vi "HighPressureVerification.vi"(8 "error in":errorcluster, 11 "S1 in":refnum<class "S1.lvclass">) -> (0 "error out":errorcluster, 3 "S1 out":refnum<class "S1.lvclass">)   [LabVIEW 2018, in "S1.lvclass"]
uses:
  S1.lvclass
  S1.lvclass/S1.ctl
  Public Controls/Outputs.ctl
  Public Controls/ReportHeader.ctl
  d2b88b60-9070-42d4-a245-a35bcc0db904.vi
  8c384891-5d03-4ede-b955-697cfc4dec26.vi
  IO/IO.lvclass
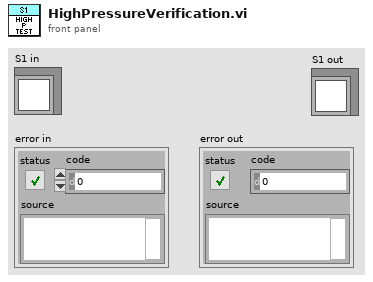
[diagram p1: front panel]
types:
  T1 = typedef "S1.lvclass/Outputs.ctl" = cluster{"LoP":bool, "HiP":bool, "Z1Vent":bool, "Z2Vent":bool, "Z3Vent":bool, "IsLidLock":bool}
  T2 = typedef "S1.lvclass/ReportHeader.ctl" = string
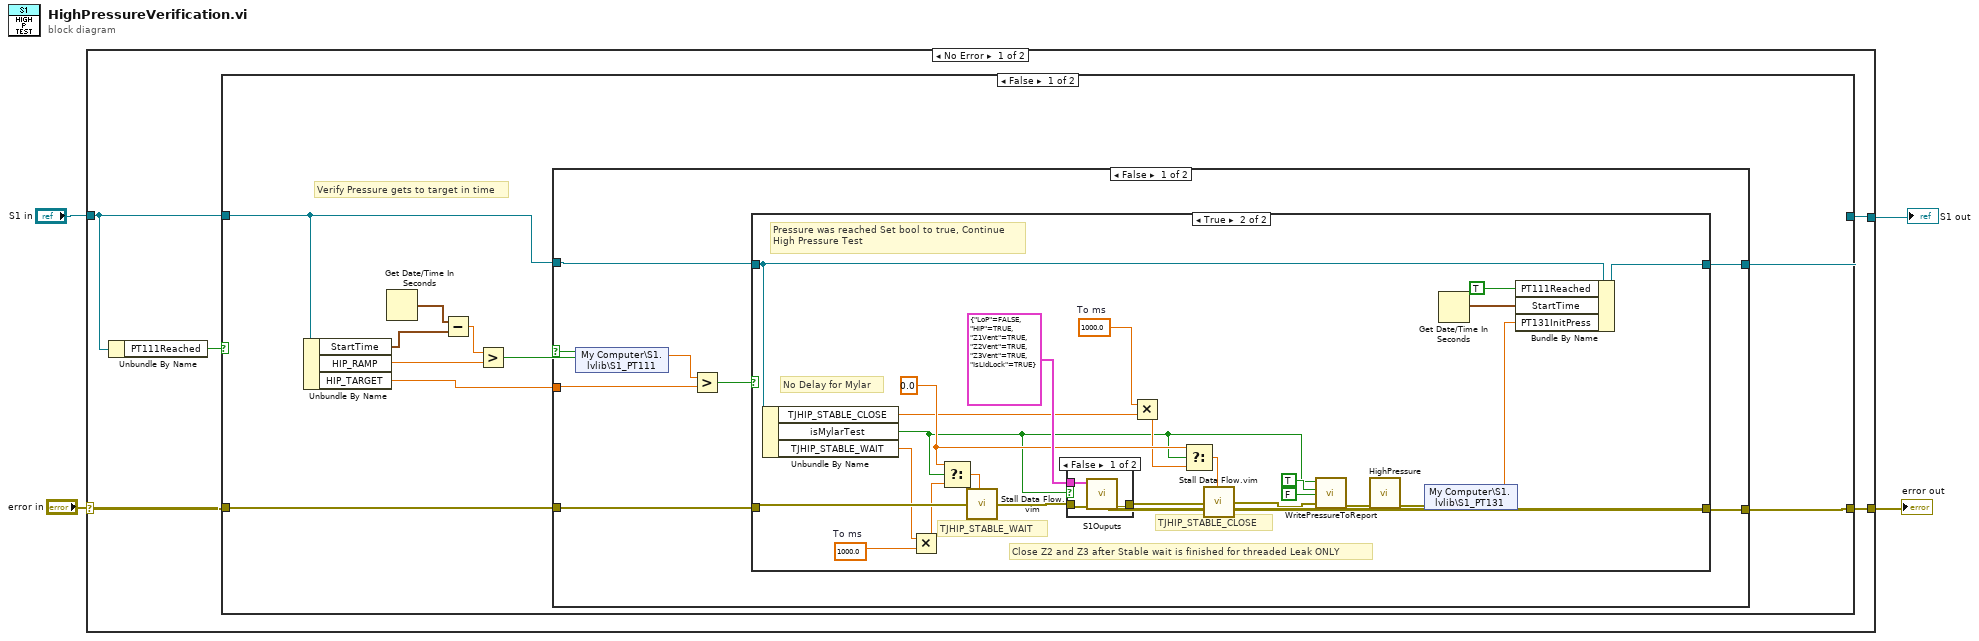
[diagram p0: block diagram]
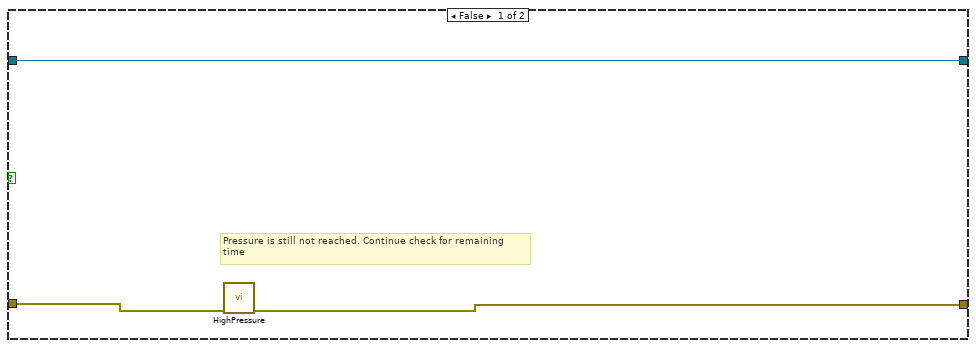
[diagram p2: hidden frame]
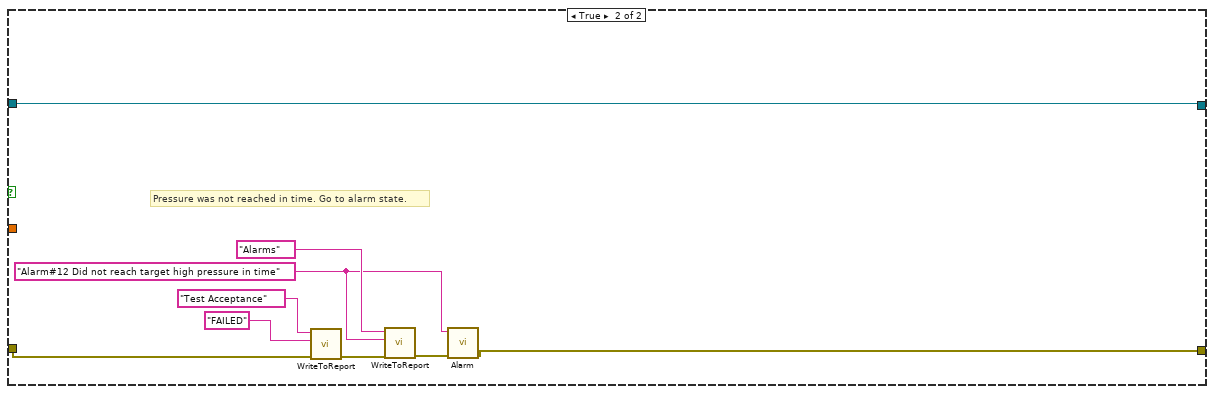
[diagram p4: hidden frame]
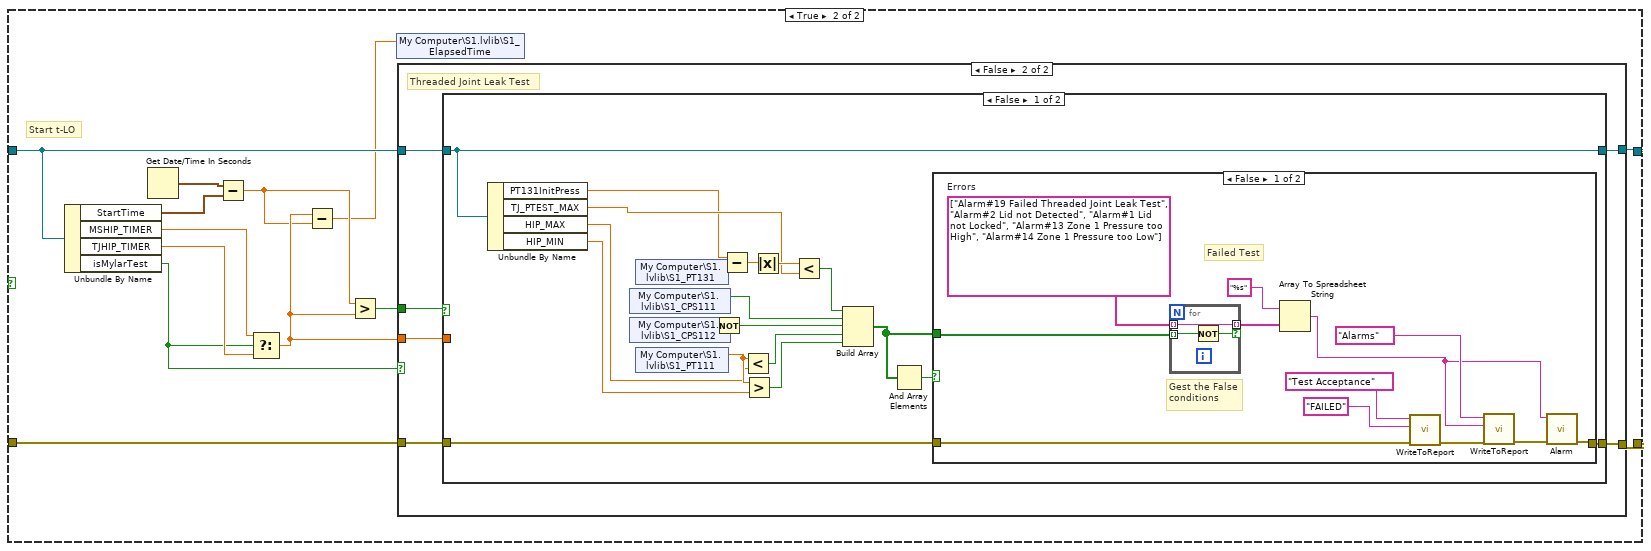
[diagram p5: hidden frame]
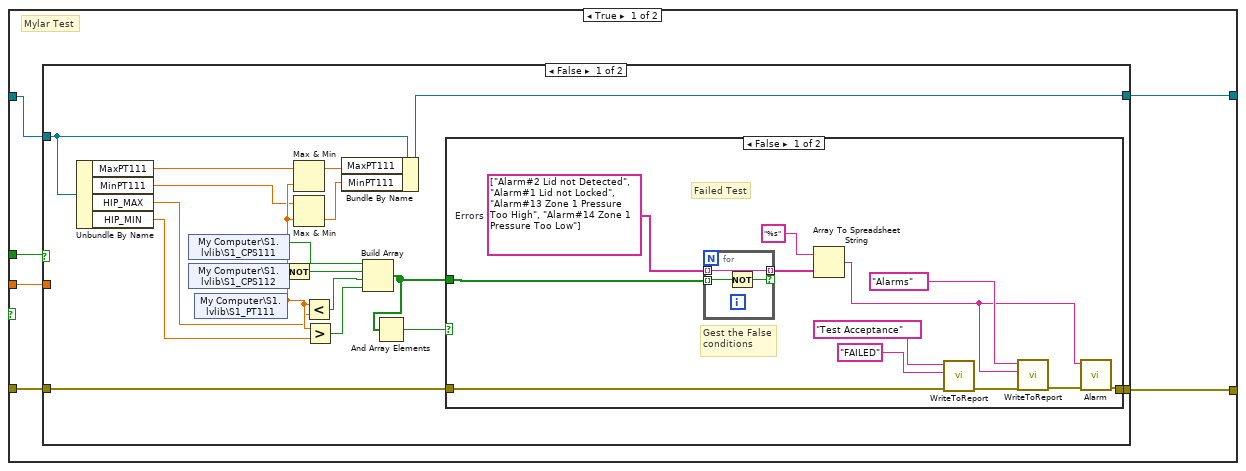
[diagram p6: hidden frame]
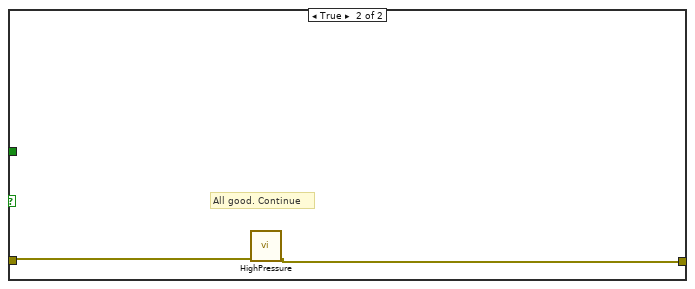
[diagram p7: hidden frame]
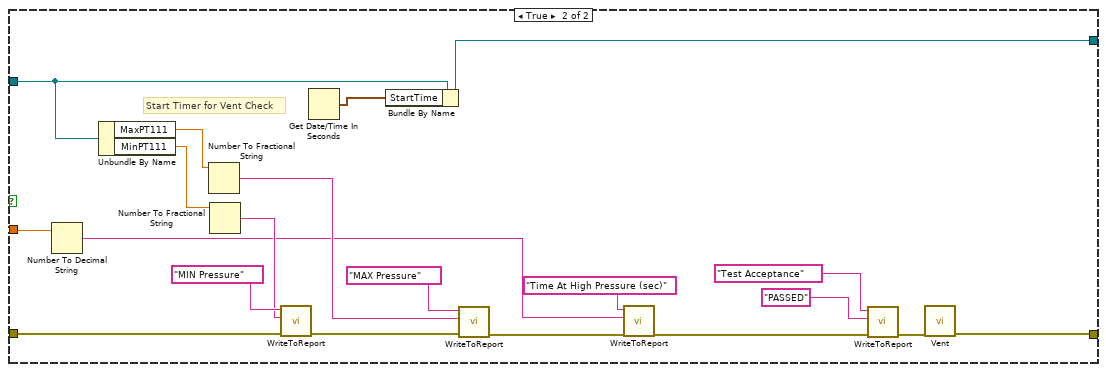
[diagram p8: hidden frame]
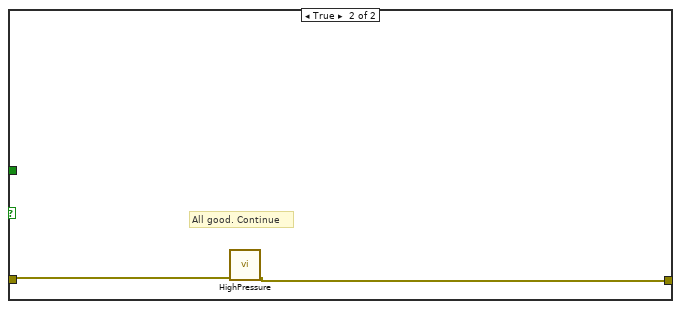
[diagram p9: hidden frame]
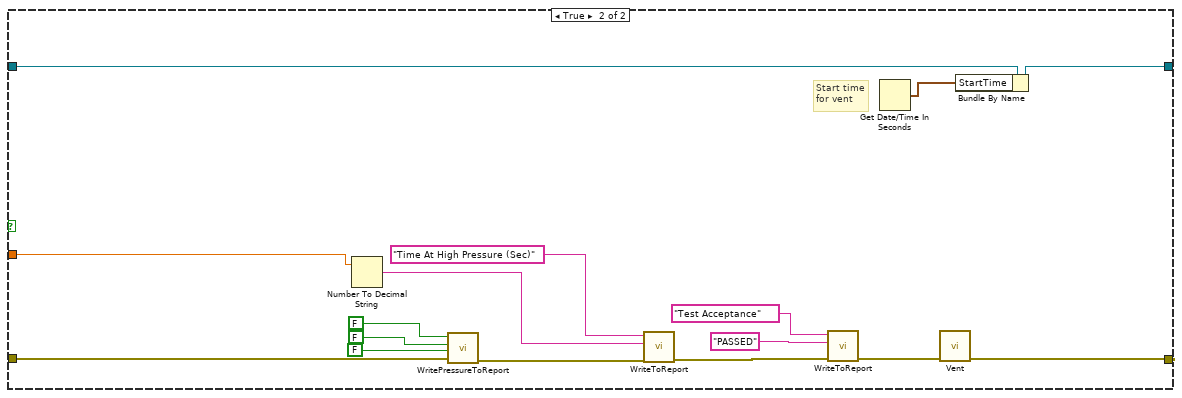
[diagram p10: hidden frame]
diagram:
  n1 = case shown="No Error" "error in" {
    selector: "error in" -> [w9 w201]
    tunnel: [w7 w201] -> w4
    tunnel: "S1 in" -> [w6 w200]
    tunnel: [w8 w200] -> w1
    frame No Error {
      n2 = Unbundle By Name(w6) -> ("PT111Reached"=w5:bool)
      n3 = case shown="False" w5 {
        tunnel: w9 -> [w17 w80]
        tunnel: [w15 w76] -> w7
        tunnel: w6 -> [w13 w75]
        tunnel: [w14 w74] -> w8
        frame False {
          # "Verify Pressure gets to target in time"
          n4 = Unbundle By Name(w13) -> ("StartTime"=w10:timestamp, "HIP_RAMP"=w12:dbl, "HIP_TARGET"=w11:dbl)
          n5 = Get Date/Time In Seconds() -> (seconds since 1Jan1904=w19:timestamp)
          n6 = Subtract(x=w19, y=w10) -> (x-y=w18:dbl)
          n7 = Greater?(x=w18, y=w12) -> (0:w16:bool)
          n8 = case shown="False" w16 {
            tunnel: w17 -> [w23 w63]
            tunnel: [w22 w61] -> w15
            tunnel: w13 -> [w25 w62]
            tunnel: [w24 w62] -> w14
            tunnel: w11 -> [w21 _]
            frame False {
              n9 = shared-variable "My Computer\\S1.lvlib\\S1_PT111"() -> (w26:dbl)  [unwired: 1 in, 1 out]
              n10 = Greater?(x=w26, y=w21) -> (0:w20:bool)
              n11 = case shown="True" w20 {
                tunnel: w25 -> [w29 w53]
                tunnel: [w29 w54] -> w24
                tunnel: w23 -> [w28 w49]
                tunnel: [w27 w47] -> w22
                frame False {
                  # "Pressure is still not reached. Continue check for remaining\ntime"
                  n12 = call "HighPressure.vi"("error in"=w28) -> ("error out"=w27:errorcluster)  [unwired: 10 in]
                }
                frame True {
                  w34 = 1000.0  # To ms
                  w35 = 0.0 ("t")
                  w43 = 1000.0  # To ms
                  # "TJHIP_STABLE_WAIT"
                  # "TJHIP_STABLE_CLOSE"
                  # "Close Z2 and Z3 after Stable wait is finished for threaded Leak ONLY"
                  # "No Delay for Mylar"
                  # "Pressure was reached Set bool to true, Continue\nHigh Pressure Test"
                  n13 = Unbundle By Name(w53) -> ("TJHIP_STABLE_CLOSE"=w33:dbl, "isMylarTest"=w30:bool, "TJHIP_STABLE_WAIT"=w45:dbl)
                  n14 = Multiply(x=w45, y=w43) -> (x*y=w44:dbl)
                  n15 = Select(t=w35, s=w30, f=w44) -> (s? t:f=w46:dbl)
                  n16 = call "Stall Data Flow.vim"("value in"=w49, "milliseconds to wait"=w46) -> ("value out"=w39:errorcluster)  [unwired: 1 out]
                  n17 = case shown="False" w30 {
                    tunnel: w39 -> [w57 w58]
                    tunnel: T1 {"LoP"=FALSE, "HiP"=TRUE, "Z1Vent"=TRUE, "Z2Vent"=TRUE, "Z3Vent"=TRUE, "IsLidLock"=TRUE} ("SIOutputs") -> [w56 _]
                    tunnel: [w55 w58] -> w37
                    frame False {
                      n18 = call "S1Ouputs.vi"("error in"=w57, "SIOutputs"=w56) -> ("error out"=w55:errorcluster)  [unwired: 9 in]
                    }
                    frame True {
                    }
                  }
                  n19 = Multiply(x=w34, y=w33) -> (x*y=w32:dbl)
                  n20 = Select(t=w35, s=w30, f=w32) -> (s? t:f=w31:dbl)
                  n21 = call "Stall Data Flow.vim"("value in"=w37, "milliseconds to wait"=w31) -> ("value out"=w36:errorcluster)  [unwired: 1 out]
                  n22 = call "WritePressureToReport.vi"("error in (no error)"=w36, "LowPressure"=FALSE, "Initial"=TRUE, "isMylarTest"=w30) -> ("error out"=w50:errorcluster)  [unwired: 7 in]
                  n23 = call "HighPressure.vi"("error in"=w50) -> ("error out"=w48:errorcluster)  [unwired: 10 in]
                  n24 = shared-variable "My Computer\\S1.lvlib\\S1_PT131"(error in=w48) -> (w40:dbl, error out=w47:errorcluster)
                  n25 = Get Date/Time In Seconds() -> (seconds since 1Jan1904=w41:timestamp)
                  n26 = Bundle By Name(cluster=w53, "PT111Reached"=TRUE ("PT111ReachedPressure"), "StartTime"=w41, "PT131InitPress"=w40) -> (w54:refnum<class "S1.lvclass">)
                }
              }
            }
            frame True {
              w60 = "Alarm#12 Did not reach target high pressure in time" ("Value")
              # "Pressure was not reached in time. Go to alarm state."
              n27 = call "WriteToReport.vi"("error in"=w63, "Value"="FAILED", "Header"=T2 "Test Acceptance") -> ("error out"=w67:errorcluster)  [unwired: 8 in]
              n28 = call "WriteToReport.vi"("error in"=w67, "Value"=w60, "Header"="Alarms") -> ("error out"=w65:errorcluster)  [unwired: 8 in]
              n29 = call "Alarm.vi"("error in"=w65, "Alarm"=w60) -> ("error out"=w61:errorcluster)  [unwired: 9 in]
            }
          }
        }
        frame True {
          # "Start t-LO"
          n30 = Unbundle By Name(w75) -> ("StartTime"=w78:timestamp, "MSHIP_TIMER"=w73:dbl, "TJHIP_TIMER"=w72:dbl, "isMylarTest"=w68:bool)
          n31 = Get Date/Time In Seconds() -> (seconds since 1Jan1904=w79:timestamp)
          n32 = Subtract(x=w79, y=w78) -> (x-y=w70:dbl)
          n33 = Select(t=w73, s=w68, f=w72) -> (s? t:f=w71:dbl)
          n34 = Subtract(x=w71, y=w70) -> (x-y=w69:dbl)
          n35 = Greater?(x=w70, y=w71) -> (0:w77:bool)
          n36 = shared-variable "My Computer\\S1.lvlib\\S1_ElapsedTime"(w69) -> ()  [unwired: 1 in, 1 out]
          n37 = case shown="False" w68 {
            tunnel: w80 -> [w85 w146]
            tunnel: [w86 w147] -> w76
            tunnel: w75 -> [w84 w145]
            tunnel: [w83 w144] -> w74
            tunnel: w77 -> [w82 w143]
            tunnel: w71 -> [w81 w142]
            frame True {
              # "Mylar Test"
              n38 = case shown="False" w82 {
                tunnel: [w104 w133] -> w86
                tunnel: w85 -> [w97 w141]
                tunnel: w84 -> [w96 w132]
                tunnel: [w93 w131] -> w83
                tunnel: w81 -> [_ w125]
                frame False {
                  n39 = Unbundle By Name(w96) -> ("MaxPT111"=w95:dbl, "MinPT111"=w91:dbl, "HIP_MAX"=w88:dbl, "HIP_MIN"=w87:dbl)
                  n40 = shared-variable "My Computer\\S1.lvlib\\S1_CPS111"() -> (w99:bool)  [unwired: 1 in, 1 out]
                  n41 = shared-variable "My Computer\\S1.lvlib\\S1_CPS112"() -> (w98:bool)  [unwired: 1 in, 1 out]
                  n42 = shared-variable "My Computer\\S1.lvlib\\S1_PT111"() -> (w94:dbl)  [unwired: 1 in, 1 out]
                  n43 = Not(x=w98) -> (.not. x?=w89:bool)
                  n44 = Max & Min(x=w95, y=w94) -> (max(x,y)=w92:dbl)  [unwired: 1 out]
                  n45 = Max & Min(x=w91, y=w94) -> (min(x,y)=w90:dbl)  [unwired: 1 out]
                  n46 = Less?(x=w94, y=w88) -> (x < y?=w103:bool)
                  n47 = Greater?(x=w94, y=w87) -> (0:w102:bool)
                  n48 = Bundle By Name(cluster=w96, "MaxPT111"=w92, "MinPT111"=w90) -> (w93:refnum<class "S1.lvclass">)
                  n49 = Build Array(w99, w89, w103, w102) -> (w100:bool[])
                  n50 = And Array Elements(Boolean array=w100) -> (logical AND=w101:bool)
                  n51 = case shown="False" w101 {
                    tunnel: w97 -> [w112 w121]
                    tunnel: [w107 w120] -> w104
                    tunnel: w100 -> [w111 _]
                    frame False {
                      w110 = string[] ["Alarm#2 Lid not Detected", "Alarm#1 Lid not Locked", "Alarm#13 Zone 1 Pressure Too High", "Alarm#14 Zone 1 Pressure Too Low"]  # Errors
                      # "Failed Test"
                      # "Gest the False\nconditions"
                      n52 = for {
                        tunnel: w111 -> [w118] mode=indexing
                        tunnel: w110 -> [w119] mode=indexing
                        tunnel: [w119] -> w109 mode=indexing if=w117
                        n53 = Not(x=w118) -> (.not. x?=w117:bool)
                      }
                      n54 = Array To Spreadsheet String(array=w109, 3:"%s" ("format string")) -> (spreadsheet string=w106:string)  [unwired: 1 in]
                      n55 = call "WriteToReport.vi"("error in"=w112, "Value"="FAILED", "Header"=T2 "Test Acceptance") -> ("error out"=w116:errorcluster)  [unwired: 8 in]
                      n56 = call "WriteToReport.vi"("error in"=w116, "Value"=w106, "Header"="Alarms") -> ("error out"=w114:errorcluster)  [unwired: 8 in]
                      n57 = call "Alarm.vi"("error in"=w114, "Alarm"=w106) -> ("error out"=w107:errorcluster)  [unwired: 9 in]
                    }
                    frame True {
                      # "All good. Continue"
                      n58 = call "HighPressure.vi"("error in"=w121) -> ("error out"=w120:errorcluster)  [unwired: 10 in]
                    }
                  }
                }
                frame True {
                  # "Start Timer for Vent Check"
                  n59 = Number To Decimal String(number=w125) -> (decimal integer string=w127:string)  [unwired: 1 in]
                  n60 = Unbundle By Name(w132) -> ("MaxPT111"=w137:dbl, "MinPT111"=w135:dbl)
                  n61 = Number To Fractional String(number=w137) -> (F-format string=w136:string)  [unwired: 3 in]
                  n62 = Number To Fractional String(number=w135) -> (F-format string=w134:string)  [unwired: 3 in]
                  n63 = call "WriteToReport.vi"("error in"=w141, "Value"=w134, "Header"="MIN Pressure") -> ("error out"=w138:errorcluster)  [unwired: 8 in]
                  n64 = Get Date/Time In Seconds() -> (seconds since 1Jan1904=w130:timestamp)
                  n65 = Bundle By Name(cluster=w132, "StartTime"=w130) -> (w131:refnum<class "S1.lvclass">)
                  n66 = call "WriteToReport.vi"("error in"=w138, "Value"=w136, "Header"="MAX Pressure") -> ("error out"=w124:errorcluster)  [unwired: 8 in]
                  n67 = call "WriteToReport.vi"("error in"=w124, "Value"=w127, "Header"="Time At High Pressure (sec)" ("decimal integer string")) -> ("error out"=w123:errorcluster)  [unwired: 8 in]
                  n68 = call "WriteToReport.vi"("error in"=w123, "Value"="PASSED", "Header"=T2 "Test Acceptance") -> ("error out"=w129:errorcluster)  [unwired: 8 in]
                  n69 = call "Vent.vi"("error in"=w129) -> ("error out"=w133:errorcluster)  [unwired: 10 in]
                }
              }
            }
            frame False {
              # "Threaded Joint Leak Test"
              n70 = case shown="False" w143 {
                tunnel: [w166 w199] -> w147
                tunnel: w146 -> [w159 w192]
                tunnel: w145 -> [w157 w198]
                tunnel: [w157 w187] -> w144
                tunnel: w142 -> [_ w184]
                frame False {
                  n71 = Unbundle By Name(w157) -> ("PT131InitPress"=w148:dbl, "TJ_PTEST_MAX"=w150:dbl, "HIP_MAX"=w155:dbl, "HIP_MIN"=w154:dbl)
                  n72 = shared-variable "My Computer\\S1.lvlib\\S1_CPS111"() -> (w161:bool)  [unwired: 1 in, 1 out]
                  n73 = shared-variable "My Computer\\S1.lvlib\\S1_CPS112"() -> (w160:bool)  [unwired: 1 in, 1 out]
                  n74 = shared-variable "My Computer\\S1.lvlib\\S1_PT131"() -> (w149:dbl)  [unwired: 1 in, 1 out]
                  n75 = shared-variable "My Computer\\S1.lvlib\\S1_PT111"() -> (w158:dbl)  [unwired: 1 in, 1 out]
                  n76 = Not(x=w160) -> (.not. x?=w156:bool)
                  n77 = Subtract(x=w148, y=w149) -> (x-y=w153:dbl)
                  n78 = Less?(x=w158, y=w155) -> (x < y?=w165:bool)
                  n79 = Greater?(x=w158, y=w154) -> (0:w164:bool)
                  n80 = Absolute Value(x=w153) -> (abs(x)=w152:dbl)
                  n81 = Less?(x=w152, y=w150) -> (x < y?=w151:bool)
                  n82 = Build Array(w151, w161, w156, w165, w164) -> (w162:bool[])
                  n83 = And Array Elements(Boolean array=w162) -> (logical AND=w163:bool)
                  n84 = case shown="False" w163 {
                    tunnel: w159 -> [w174 w183]
                    tunnel: [w168 w182] -> w166
                    tunnel: w162 -> [w173 _]
                    frame False {
                      w172 = string[] ["Alarm#19 Failed Threaded Joint Leak Test", "Alarm#2 Lid not Detected", "Alarm#1 Lid not Locked", "Alarm#13 Zone 1 Pressure too High", "Alarm#14 Zone 1 Pressure too Low"]  # Errors
                      # "Failed Test"
                      # "Gest the False\nconditions"
                      n85 = for {
                        tunnel: w173 -> [w180] mode=indexing
                        tunnel: w172 -> [w181] mode=indexing
                        tunnel: [w181] -> w171 mode=indexing if=w179
                        n86 = Not(x=w180) -> (.not. x?=w179:bool)
                      }
                      n87 = Array To Spreadsheet String(array=w171, 3:"%s" ("format string")) -> (spreadsheet string=w169:string)  [unwired: 1 in]
                      n88 = call "WriteToReport.vi"("error in"=w174, "Value"="FAILED", "Header"=T2 "Test Acceptance") -> ("error out"=w178:errorcluster)  [unwired: 8 in]
                      n89 = call "WriteToReport.vi"("error in"=w178, "Value"=w169, "Header"="Alarms") -> ("error out"=w176:errorcluster)  [unwired: 8 in]
                      n90 = call "Alarm.vi"("error in"=w176, "Alarm"=w169) -> ("error out"=w168:errorcluster)  [unwired: 9 in]
                    }
                    frame True {
                      # "All good. Continue"
                      n91 = call "HighPressure.vi"("error in"=w183) -> ("error out"=w182:errorcluster)  [unwired: 10 in]
                    }
                  }
                }
                frame True {
                  # "Start time\nfor vent"
                  n92 = Number To Decimal String(number=w184) -> (decimal integer string=w193:string)  [unwired: 1 in]
                  n93 = call "WritePressureToReport.vi"("error in (no error)"=w192, "LowPressure"=FALSE, "Initial"=FALSE, "isMylarTest"=FALSE) -> ("error out"=w191:errorcluster)  [unwired: 7 in]
                  n94 = call "WriteToReport.vi"("error in"=w191, "Value"=w193, "Header"="Time At High Pressure (Sec)" ("decimal integer string")) -> ("error out"=w190:errorcluster)  [unwired: 8 in]
                  n95 = call "WriteToReport.vi"("error in"=w190, "Value"="PASSED", "Header"=T2 "Test Acceptance") -> ("error out"=w189:errorcluster)  [unwired: 8 in]
                  n96 = Get Date/Time In Seconds() -> (seconds since 1Jan1904=w186:timestamp)
                  n97 = call "Vent.vi"("error in"=w189) -> ("error out"=w199:errorcluster)  [unwired: 10 in]
                  n98 = Bundle By Name(cluster=w198, "StartTime"=w186) -> (w187:refnum<class "S1.lvclass">)
                }
              }
            }
          }
        }
      }
    }
    frame Error {
    }
  }
  "error out" <- w4
  "S1 out" <- w1
